vi "sedSpectrometer_registerCallback_logEvent_.vi"(8 "error in (no error)":errorcluster, 10 "skipOld":bool, 11 "handle":i32) -> (0 "error out":errorcluster, 3 "function return":i32)   [LabVIEW 2016, in "SALLV_sedSpectrometer.lvlib"]
doc: "int sedSpectrometer_shm_registerCallback_logeventLV(int handle, bool skipOld);"
uses:
  SALLV_sedSpectrometer.lvlib
  SALLV_sedSpectrometer.so
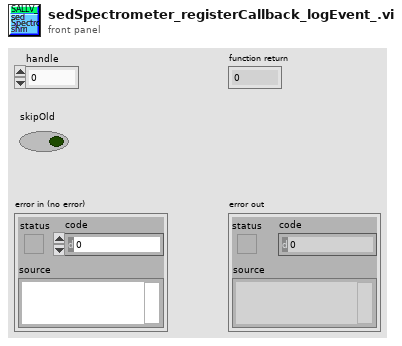
[diagram p1: front panel]
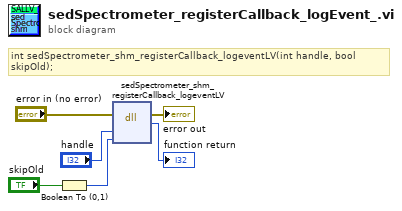
[diagram p0: block diagram]
diagram:
  # "int sedSpectrometer_shm_registerCallback_logeventLV(int handle, bool skipOld);"
  n1 = Boolean To (0,1)(Boolean="skipOld") -> (0, 1=w3:i16)
  n2 = dll-call lib="home/harini/TCS/SALLV_sedSpectrometer/SALLV_sedSpectrometer.*" fn="sedSpectrometer_shm_registerCallback_logeventLV"(error in="error in (no error)", "handle"="handle", "skipOld"=w3) -> (error out=→"error out":errorcluster, →"function return":i32)  [unwired: 4 in, 1 out]
